vi "Get Set Hostname.vi"(8 "Error In":errorcluster, 9 "Set":bool, 10 "Hostname":string, 11 "Install LV Data":T1={"SSH Session"=refnum, "Status Log"="", "Detailed Log"="", "Credentials"={"Hostname or IP"="192.168.7.2", "Username"="root", "Password"=""}, "Target Info"={"OS Version"="", "CPU"="", "Systemd Version"="", "Internet Access"=FALSE, "Device Type"="", "LV Installed Ver"="", "LV Available Ver"="", "LV Upgrade Available"=FALSE, "Hostname"="", "NIC Info"=[]}, "Reboot Required?"=FALSE}) -> (0 "Error Out":errorcluster, 2 "Hostname":string, 3 "Install LV Data":T1={"SSH Session"=refnum, "Status Log"="", "Detailed Log"="", "Credentials"={"Hostname or IP"="192.168.7.2", "Username"="root", "Password"=""}, "Target Info"={"OS Version"="", "CPU"="", "Systemd Version"="", "Internet Access"=FALSE, "Device Type"="", "LV Installed Ver"="", "LV Available Ver"="", "LV Upgrade Available"=FALSE, "Hostname"="", "NIC Info"=[]}, "Reboot Required?"=FALSE})   [LabVIEW 2020, in "LMH-LINX.lvlib"]
uses:
  LMH-LINX.lvlib
  Install LV Data.ctl
  Target Info.ctl
  NIC Info.ctl
  NIC Mode.ctl
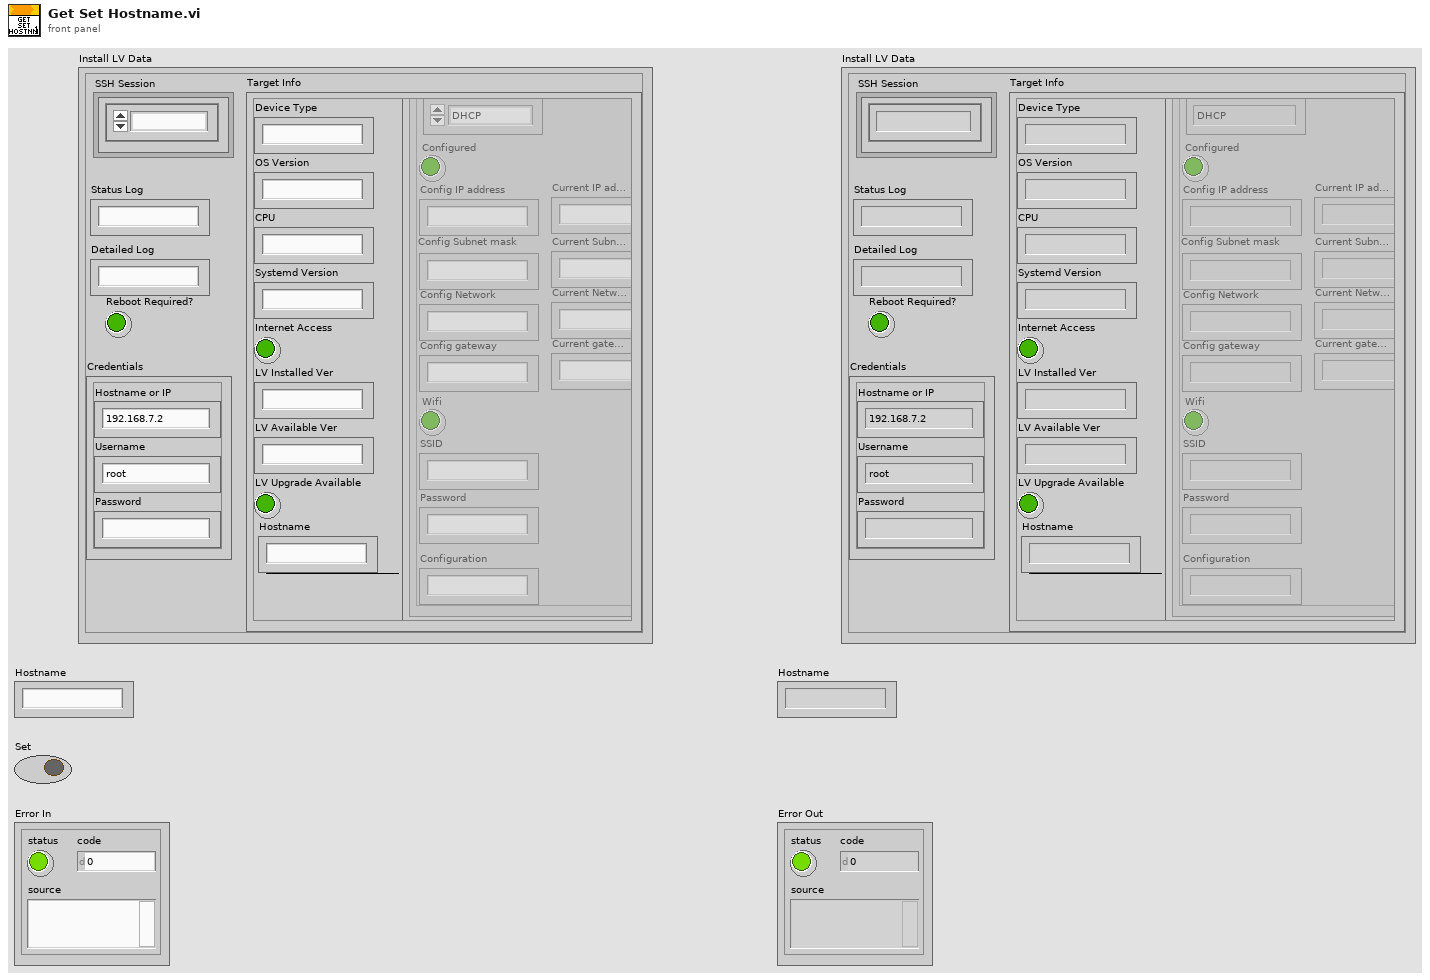
[diagram p1: front panel]
types:
  T1 = typedef "LMH-LINX.lvlib/Install LV Data.ctl" = cluster{"SSH Session":refnum<k1>, "Status Log":string, "Detailed Log":string, "Credentials":cluster{"Hostname or IP":string, "Username":string, "Password":string}, "Target Info":T2, "Reboot Required?":bool}
  T2 = typedef "LMH-LINX.lvlib/Target Info.ctl" = cluster{"OS Version":string, "CPU":string, "Systemd Version":string, "Internet Access":bool, "Device Type":string, "LV Installed Ver":string, "LV Available Ver":string, "LV Upgrade Available":bool, "Hostname":string, "NIC Info":T3[]}
  T3 = typedef "LMH-LINX.lvlib/NIC Info.ctl" = cluster{"Name":string, "NIC Mode":T4, "Configured":bool, "Config IP address":string, "Config Subnet mask":string, "Config Network":string, "Config gateway":string, "Wifi":bool, "SSID":string, "Password":string, "Configuration":string, "Current IP address":string, "Current Subnet mask":string, "Current gateway":string, "Current Network":string}
  T4 = typedef "LMH-LINX.lvlib/NIC Mode.ctl" = enum16{"DHCP", "Static", "Loopback"}
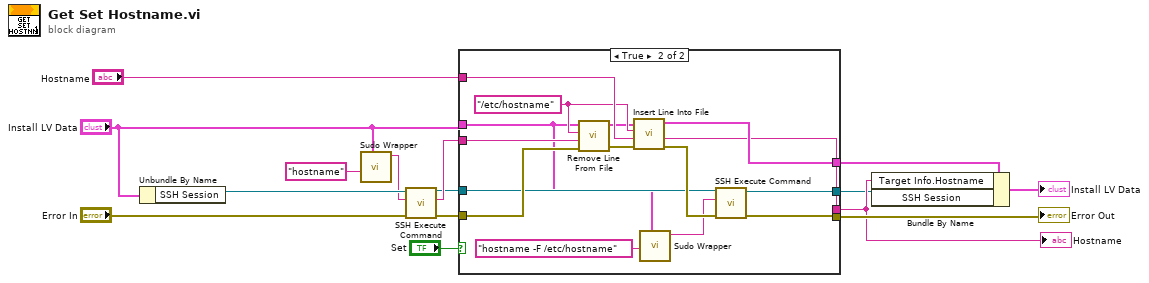
[diagram p0: block diagram]
diagram:
  n1 = Unbundle By Name("Install LV Data") -> ("SSH Session"=w11:refnum<k1>)
  n2 = call "Sudo Wrapper.vi"("Install LV Data"="Install LV Data", "comand string"="hostname" ("Command")) -> ("combined command string"=w2:string)  [unwired: 9 in]
  n3 = call "SSH Execute Command.vi"("Error In"="Error In", "Command"=w2, "SSH Session"=w11) -> ("Error Out"=w13:errorcluster, "Std Out"=w9:string, "SSH Session"=w5:refnum<k1>)  [unwired: 6 in]
  n4 = case shown="True" "Set" {
    tunnel: "Hostname" -> [_ w34]
    tunnel: [w16 w33] -> w8
    tunnel: [w19 w25] -> w14
    tunnel: w9 -> [w18 w29]
    tunnel: w13 -> [w19 w28]
    tunnel: [w18 w27] -> w7
    tunnel: "Install LV Data" -> [w16 w20]
    tunnel: w5 -> [w17 w24]
    tunnel: [w17 w23] -> w4
    frame False {
    }
    frame True {
      w32 = "/etc/hostname" ("File Path")
      n5 = call "Remove Line From File.vi"("Error In"=w28, "Line"=w29, "File Path"=w32, "Install LV Data"=w20) -> ("Error Out"=w31:errorcluster, "Install LV Data"=w30:T1)  [unwired: 4 in, 2 out]
      n6 = call "Insert Line Into File.vi"("Error In"=w31, "Line"=w34, "File Path"=w32, "Install LV Data"=w30) -> ("Error Out"=w26:errorcluster, "Log"=w27:string, "Install LV Data"=w33:T1)  [unwired: 4 in, 1 out]
      n7 = call "Sudo Wrapper.vi"("Install LV Data"=w20, "comand string"="hostname -F /etc/hostname" ("File Path")) -> ("combined command string"=w21:string)  [unwired: 9 in]
      n8 = call "SSH Execute Command.vi"("Error In"=w26, "Command"=w21, "SSH Session"=w24) -> ("Error Out"=w25:errorcluster, "SSH Session"=w23:refnum<k1>)  [unwired: 6 in, 1 out]
    }
  }
  "Hostname" <- w7
  "Error Out" <- w14
  n9 = Bundle By Name(cluster=w8, "Target Info.Hostname"=w7, "SSH Session"=w4) -> (→"Install LV Data":T1)
